vi "EDS test 01.vi"() -> ()   [LabVIEW 2020]
uses:
  <vilib>/Instr/_visa.llb/VISA Configure Serial Port (Instr).vi
panel:
  out "read buffer":string
  out "output 2":dbl
  out "output 1":dbl
  in  "stop":bool
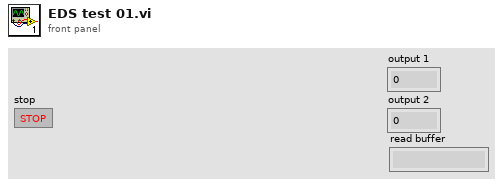
[diagram p1: front panel]
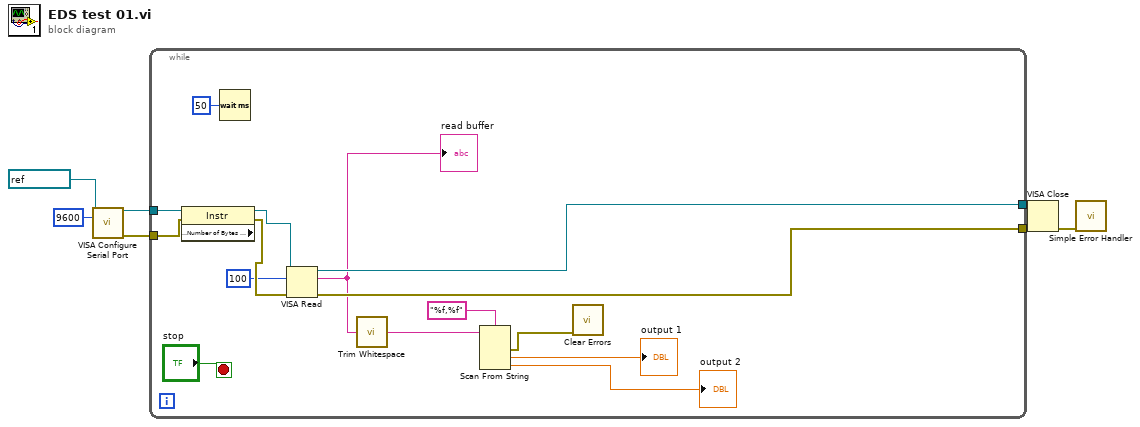
[diagram p0: block diagram]
diagram:
  n1 = call-poly "VISA Configure Serial Port"("VISA resource name"=refnum<visa-resource-name> "COM3", "baud rate (9600)"=u32 9600) -> ("VISA resource name out"=w5:refnum<visa-resource-name>, "error out"=w4:errorcluster)  [unwired: 12 in]
  n2 = while {
    tunnel: w5 -> [w22]
    tunnel: w4 -> [w21]
    tunnel: [w15] -> w3
    tunnel: [w16] -> w2
    stop <- "stop" stop-if-true
    n3 = property class="Instr" props=["Serial Settings:Number of Bytes at Serial Port"](reference=w22, error in=w21) -> (reference out=w17:refnum<visa-resource-name>, error out=w18:errorcluster)  [unwired: 1 out]
    n4 = Wait (ms)(milliseconds to wait=u32 50) -> ()  [unwired: 1 out]
    n5 = VISA Read(VISA resource name=w17, byte count=u32 100, error in (no error)=w18) -> (VISA resource name out=w15:refnum<visa-resource-name>, read buffer=w14:string, error out=w16:errorcluster)  [unwired: 1 out]
    "read buffer" <- w14
    n6 = call <vilib>:"Trim Whitespace.vi"("string"=w14) -> ("trimmed string"=w13:string)  [unwired: 1 in]
    n7 = Scan From String(format string="%f,%f", input string=w13) -> (error out=w9:errorcluster, output 1=→"output 1":dbl, output 2=→"output 2":dbl)  [unwired: 4 in, 2 out]
    n8 = call <vilib>:"Clear Errors.vi"("error in (no error)"=w9) -> ()  [unwired: 5 in, 2 out]
  }
  n9 = VISA Close(VISA resource name=w3, error in (no error)=w2) -> (error out=w1:errorcluster)
  n10 = call <vilib>:"Simple Error Handler.vi"("error in (no error)"=w1) -> ()  [unwired: 4 in, 5 out]
